vi "Adquisicion de voltaje - Velocidad - corriente y VFD.vi"() -> ()   [LabVIEW 2019]
uses:
  <vilib>/NI/Modbus Library/API/Wrapper/Create Serial Master.vi
  <vilib>/Waveform/WDTOps.llb/WDT Append Waveforms DBL.vi
  <vilib>/NI/Modbus Library/API/Master/Modbus Master.lvclass
  <vilib>/NI/Modbus Library/API/Wrapper/API Main.lvlib
panel:
  in  "VFD":bool
  in  "Frequency":dbl(knob) step=1.0 scale=0.0..75.0
  in  "stop":bool
  in  "Baud rate":u32=9600
  in  "Puerto":refnum<visa-resource-name>
  out "Velocidad medida (rpm)":dbl
  out "Frecuencia":dbl
  in  "Stop":bool=TRUE
  in  "Control de Caragas":T1(ring)
  in  "Motor a analizar":dbl
  out "Torque":dbl
  out "Torque":dbl(knob) scale=-10.0..10.0
  out "Corriente generado":dynamicdata(graph)
  out "Corriente":dbl
  out "Voltaje":dbl
  out "Corriente RMS":dbl(knob) scale=0.0..2.0
  out "Voltaje generado":dynamicdata(graph)
  out "Voltaje RMS":dbl(knob) scale=0.0..230.0
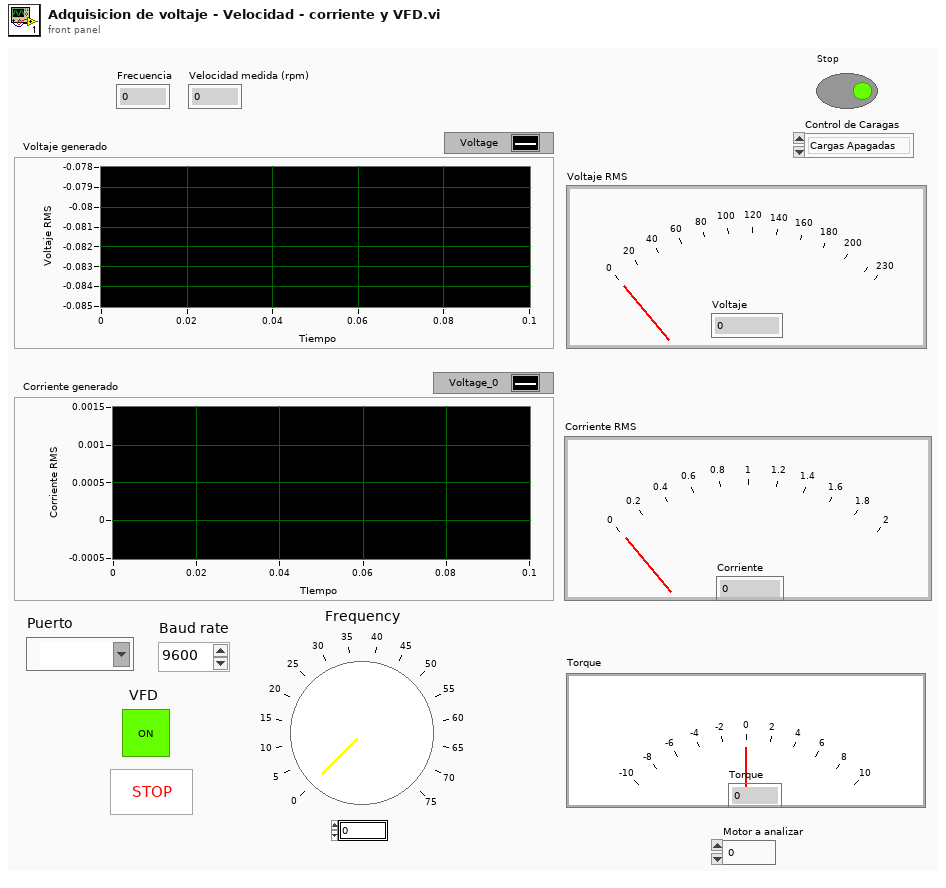
[diagram p1: front panel]
types:
  T1 = enum16{"Cargas Apagadas", "Activar Primer Carga", "Activar Segunda Carga", "Activar Ambas Cargas"}
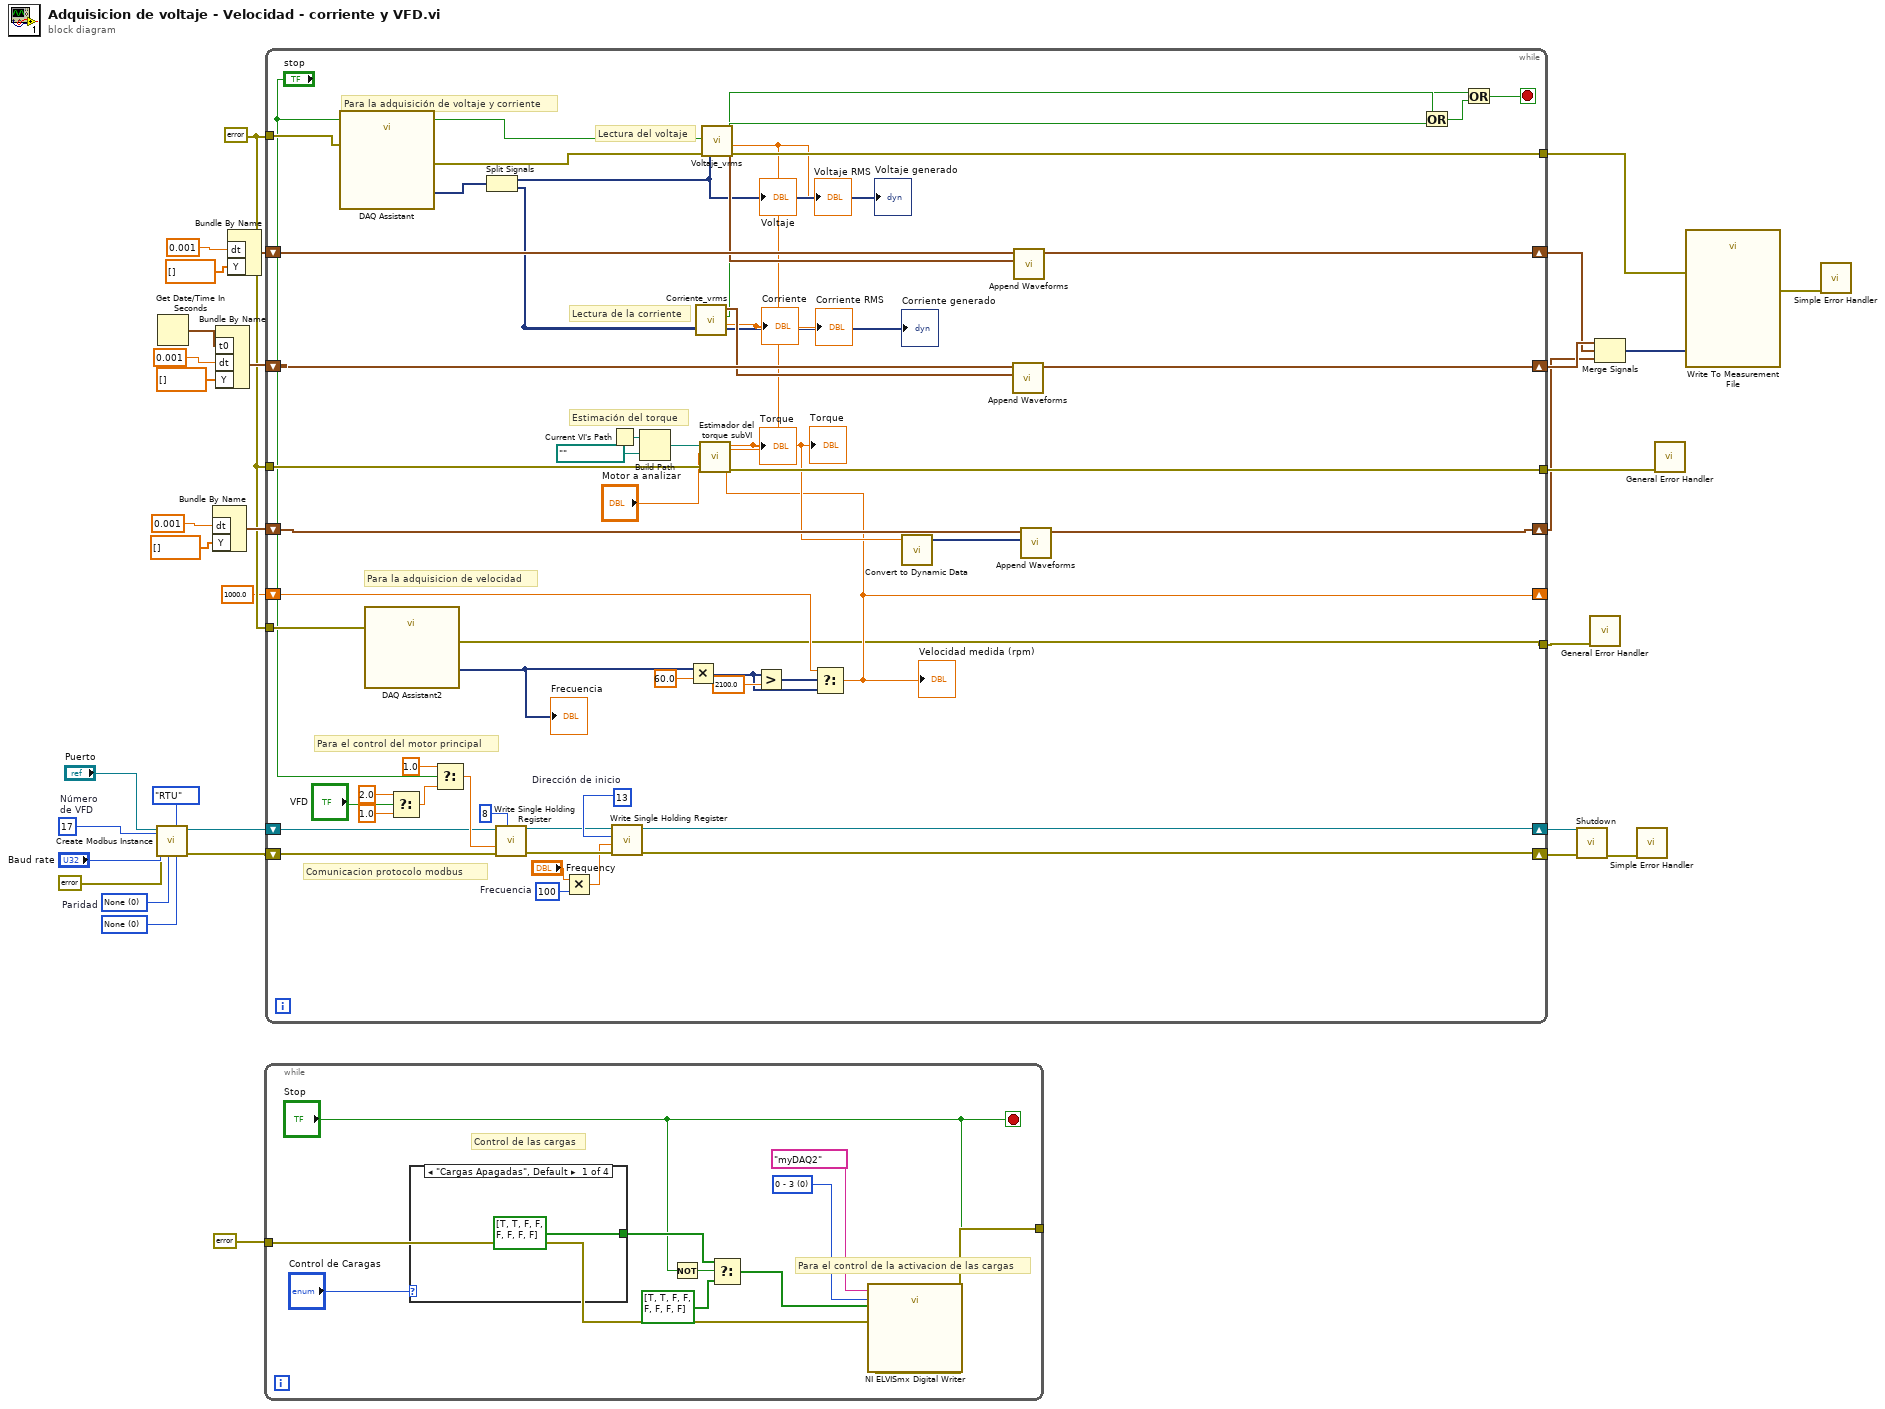
[diagram p0: block diagram]
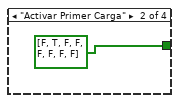
[diagram p2: hidden frame]
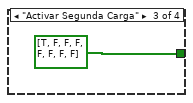
[diagram p3: hidden frame]
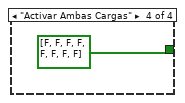
[diagram p4: hidden frame]
diagram:
  w7 = u16 0 items=["None", "Odd", "Even", "Mark", "Space"]  # Paridad
  w8 = u16 0 items=["None", "XON/XOFF", "RTS/CTS", "XON/XOFF & RTS/CTS", "DTR/DSR", "XON/XOFF & DTR/DSR"] ("flow control (none)")
  w6 = u8 17  # Número de VFD
  w15 = errorcluster {"status"=FALSE, "code"=0, "source"=""} ("error in")
  n1 = call-poly <vilib>:"Create Modbus Instance.vi"("flow control (none)"=w8, "serial type"=enum16{"RTU", "ASCII"}."RTU", "parity (even)"=w7, "unit ID"=w6, "error in"=errorcluster {"status"=FALSE, "code"=0, "source"=""}, "baud rate"="Baud rate", "VISA resource name"="Puerto") -> ("error out"=w4:errorcluster, "serial master instance"=w5:refnum<class "Modbus Master.lvclass">)  [unwired: 3 in]
  n2 = Get Date/Time In Seconds() -> (seconds since 1Jan1904=w31:timestamp)
  n3 = Bundle By Name("dt"=0.001, "Y"=dbl[] []) -> (w21:waveform(dbl))  [unwired: 1 in]
  n4 = Bundle By Name("t0"=w31, "dt"=0.001, "Y"=dbl[] []) -> (w30:waveform(dbl))  [unwired: 1 in]
  n5 = Bundle By Name("dt"=0.001, "Y"=dbl[] []) -> (w25:waveform(dbl))  [unwired: 1 in]
  n6 = while {
    tunnel: errorcluster {"status"=FALSE, "code"=0, "source"=""} ("error in") -> [w36]
    tunnel: [w35] -> _
    stop <- "Stop" stop-if-true
    w37 = u16 0 items=["0 - 3", "4 - 7", "0 - 7"] ("myDAQ Lines to Write")
    # "Control de las cargas"
    # "Para el control de la activacion de las cargas"
    n7 = case shown="\"Cargas Apagadas\", Default" "Control de Caragas" {
      tunnel: [bool[] [TRUE, TRUE, FALSE, FALSE, FALSE, FALSE, FALSE, FALSE] ("DO Lines") bool[] [FALSE, TRUE, FALSE, FALSE, FALSE, FALSE, FALSE, FALSE] ("DO Lines") bool[] [TRUE, FALSE, FALSE, FALSE, FALSE, FALSE, FALSE, FALSE] ("DO Lines") bool[] [FALSE, FALSE, FALSE, FALSE, FALSE, FALSE, FALSE, FALSE] ("DO Lines")] -> w41
      frame "Cargas Apagadas", Default {
      }
      frame "Activar Primer Carga" {
      }
      frame "Activar Segunda Carga" {
      }
      frame "Activar Ambas Cargas" {
      }
    }
    n8 = Not(x="Stop") -> (.not. x?=w42:bool)
    n9 = Select(t=w41, s=w42, f=bool[] [TRUE, TRUE, FALSE, FALSE, FALSE, FALSE, FALSE, FALSE] ("DO Lines")) -> (s? t:f=w38:bool[])
    n10 = call "NI ELVISmx Digital Writer"("Device Name"=tag "myDAQ2", "myDAQ Lines to Write"=w37, "Stop"="Stop", "DO Lines"=w38, "error in"=w36) -> ("error out"=w35:errorcluster)  [unwired: 14 in]
  }
  n11 = while {
    tunnel: w15 -> [w69]
    shift-right: [w102] -> w29
    shift-left: w30 -> [w99]
    tunnel: [w101] -> w17
    shift-right: [w100] -> w28
    shift-left: w25 -> [w98]
    tunnel: w15 -> [w85]
    tunnel: [w83] -> w24
    shift-right: [w81] -> w20
    shift-left: w21 -> [w80]
    tunnel: w15 -> [w66]
    tunnel: [w68] -> w13
    shift-right: [w72] -> _
    shift-left: 1000.0 -> [w73]
    shift-right: [w49] -> w2
    shift-left: w5 -> [w52]
    shift-right: [w50] -> w1
    shift-left: w4 -> [w51]
    stop <- w97 stop-if-true
    w57 = u16 100  # Frecuencia
    w64 = u16 13  # Dirección de inicio
    # "Comunicacion protocolo modbus"
    # "Para el control del motor principal"
    # "Para la adquisicion de velocidad"
    # "Para la adquisición de voltaje y corriente"
    # "Estimación del torque"
    # "Lectura de la corriente"
    # "Lectura del voltaje"
    n12 = call "DAQ Assistant"("error in"=w69) -> ("data"=w71:dynamicdata, "error out"=w70:errorcluster)  [unwired: 16 in, 1 out]
    n13 = call "DAQ Assistant2"("error in"=w66) -> ("data"=w67:dynamicdata, "error out"=w68:errorcluster)  [unwired: 16 in, 1 out]
    "Frecuencia" <- w67
    n14 = Select(t=2.0, s="VFD", f=1.0) -> (s? t:f=w54:dbl)
    n15 = Select(t=1.0, s="stop", f=w54) -> (s? t:f=w55:dbl)
    n16 = Split Signals(w71) -> (w95:dynamicdata, w89:dynamicdata)  [unwired: 2 in]
    "Voltaje generado" <- w95
    "Corriente generado" <- w89
    n17 = call-dynamic "Write Single Holding Register.vi"("error in"=w51, "register to write"=w55, "address"=u16 8 ("Start"), "Modbus master in"=w52) -> ("error out"=w62:errorcluster, "Modbus master out"=w63:refnum<class "Modbus Master.lvclass">)  [unwired: 6 in]
    n18 = Multiply(x="Frequency", y=w57) -> (x*y=w56:dbl)
    n19 = Current VI's Path() -> (path=w88:path)
    n20 = call-dynamic "Write Single Holding Register.vi"("error in"=w62, "register to write"=w56, "address"=w64, "Modbus master in"=w63) -> ("error out"=w50:errorcluster, "Modbus master out"=w49:refnum<class "Modbus Master.lvclass">)  [unwired: 6 in]
    n21 = Build Path(base path=w88, name or relative path=path "") -> (appended path=w86:path)
    n22 = Multiply(x=w67, y=60.0) -> (x*y=w74:dynamicdata)
    n23 = call "Corriente_vrms.vi"("Dynamic Data"=w89) -> ("Scalar"=→"Corriente RMS" →"Corriente":dbl, "Boolean"=w92:bool, "Waveform"=w94:waveform(dbl))  [unwired: 8 in]
    n24 = call "Voltaje_vrms.vi"("error in (no error)"=w70, "data"=w95) -> ("error out"=w101:errorcluster, "Scalar"=w84:dbl, "Waveform"=w96:waveform(dbl), "Boolean"=w91:bool)  [unwired: 6 in]
    "Voltaje RMS" <- w84
    "Voltaje" <- w84
    n25 = Greater?(x=w74, y=2100.0) -> (0:w75:dynamicdata)
    n26 = Select(t=w73, s=w75, f=w74) -> (s? t:f=w72:dbl)
    "Velocidad medida (rpm)" <- w72
    n27 = call "Estimador del torque subVI.vi"("Real"=w84, "error in (no error)"=w85, "Real 2"=w72, "Real 3"="Motor a analizar", "appended path"=w86) -> ("error out"=w83:errorcluster, "Numeric"=w78:dbl)  [unwired: 5 in]
    "Torque" <- w78
    "Torque" <- w78
    n28 = call "Convert to Dynamic Data"("Double"=w78) -> ("Dynamic Data Type"=w79:dynamicdata)  [unwired: 3 in]
    n29 = call-poly <vilib>:"Append Waveforms.vi"("waveform B"=w94, "waveform A"=w99) -> ("waveform out"=w102:waveform(dbl))  [unwired: 8 in, 1 out]
    n30 = call-poly <vilib>:"Append Waveforms.vi"("waveform B"=w96, "waveform A"=w98) -> ("waveform out"=w100:waveform(dbl))  [unwired: 8 in, 1 out]
    n31 = call-poly <vilib>:"Append Waveforms.vi"("waveform B"=w79, "waveform A"=w80) -> ("waveform out"=w81:waveform(dbl))  [unwired: 8 in, 1 out]
    n32 = Or(x=w91, y=w92) -> (x .or. y?=w90:bool)
    n33 = Or(x="stop", y=w90) -> (x .or. y?=w97:bool)
  }
  n34 = call-dynamic "Shutdown.vi"("error in"=w1, "Modbus master in"=w2) -> ("error out"=w3:errorcluster)  [unwired: 9 in]
  n35 = call <vilib>:"General Error Handler.vi"("error in (no error)"=w13) -> ()  [unwired: 10 in, 5 out]
  n36 = Merge Signals(w29, w28, w20) -> (w19:dynamicdata)
  n37 = call <vilib>:"Simple Error Handler.vi"("error in (no error)"=w3) -> ()  [unwired: 4 in, 5 out]
  n38 = call <vilib>:"General Error Handler.vi"("error in (no error)"=w24) -> ()  [unwired: 10 in, 5 out]
  n39 = call "Write To Measurement File"("Signals"=w19, "error in (no error)"=w17) -> ("error out"=w18:errorcluster)  [unwired: 15 in, 2 out]
  n40 = call <vilib>:"Simple Error Handler.vi"("error in (no error)"=w18) -> ()  [unwired: 4 in, 5 out]
